vi "Send image to image display controller-subvi.vi"(0 "Image":T1, 1 "Window Title":string, 2 "Window Number":i32, 3 "error in":errorcluster, 4 "Image Type":T2 items=["Grayscale (U8)", "Grayscale (I16)", "Grayscale (SGL)", "Complex (CSG)", "RGB (U32)", "HSL (U32)", "RGB (U64)", "Grayscale (U16)"], 5 "Start display controller?":bool, 6 "Quit display controller?":bool) -> (7 "Image Out":T1, 10 "error out":errorcluster)   [LabVIEW 2014]
doc: "Uses a user event to send an image to Image Display controller which is running in a separate thread, if both Start and Quit inputs are false.\n\nStart = TRUE launches the display controller as a separate thread; all other inputs are ignored.\n\nQuit = TRUE sends a message to the controller telling is to close the display windows and quit."
uses:
  <vilib>/vision/Image Controls.llb/IMAQ Image.ctl
  ctt's/Image to Display event.ctt
  Globals/Initilize Globals.vi
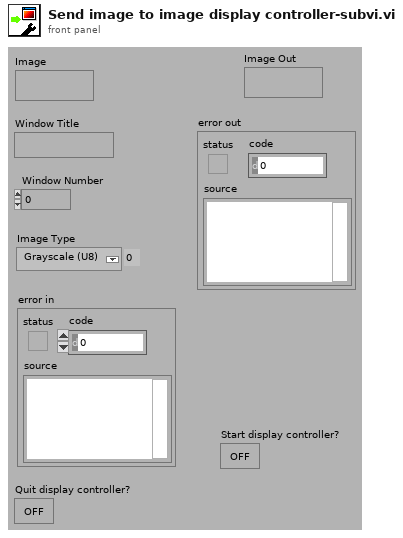
[diagram p1: front panel]
types:
  T1 = typedef "IMAQ Image.ctl" = refnum<image>
  T2 = typedef "Image Type" = u32
  T3 = typedef "Image to Display event.ctt" = cluster{"Image":T1, "Window Title":string, "Window Number":i32, "Image Type":T2, "Quit display controller?":bool}
  T4 = enum32{"Invalid", "Standard", "Closed", "Hidden", "Minimized", "Maximized"}
  T5 = enum32{"Bad", "Idle", "Run top level", "Running"}
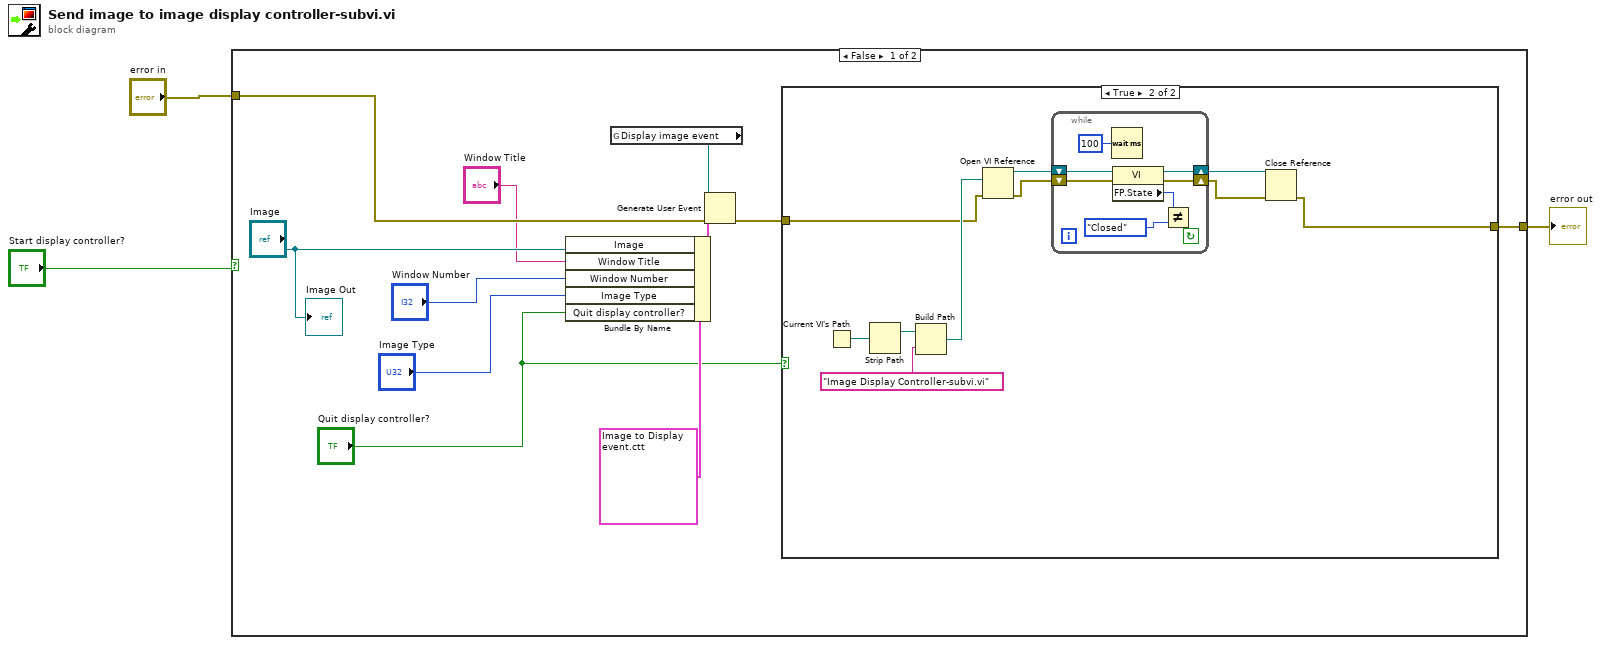
[diagram p0: block diagram]
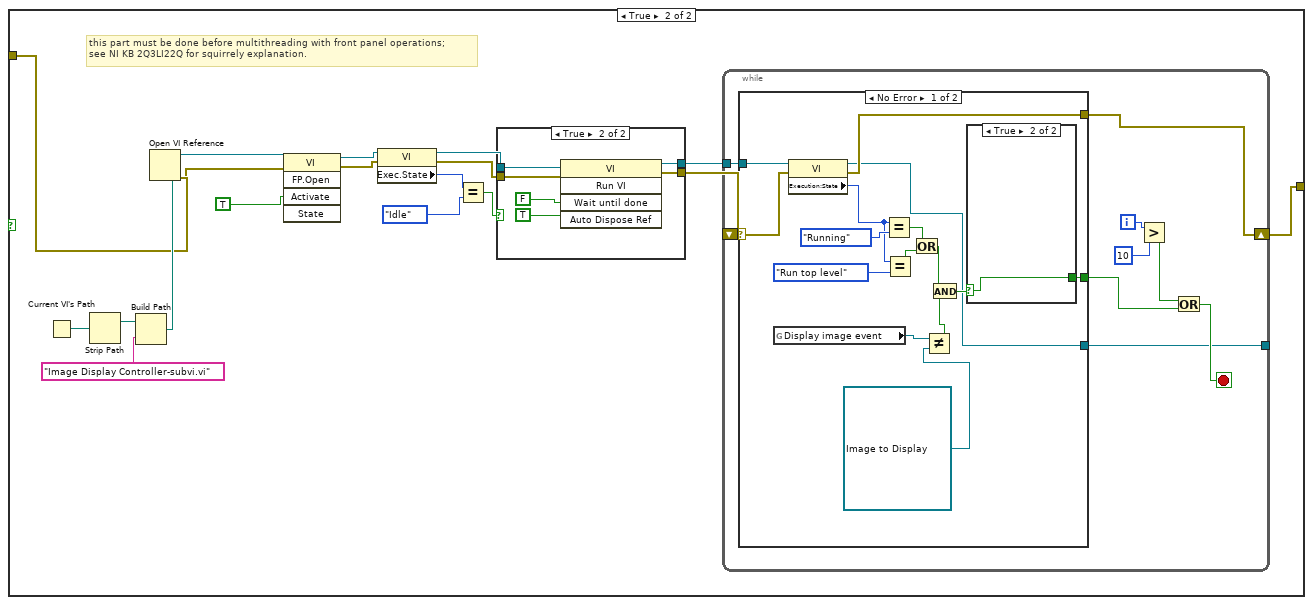
[diagram p3: hidden frame]
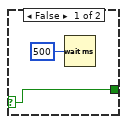
[diagram p5: hidden frame]
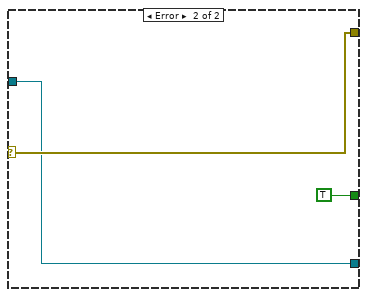
[diagram p6: hidden frame]
diagram:
  n1 = case shown="False" "Start display controller?" {
    tunnel: [w4 w46] -> w3
    tunnel: "error in" -> [w13 w47]
    frame False {
      n2 = Bundle By Name(cluster=T3 {"Image"=refnum, "Window Title"="", "Window Number"=0, "Image Type"=0, "Quit display controller?"=FALSE} ("event data"), "Image"="Image", "Window Title"="Window Title", "Window Number"="Window Number", "Image Type"="Image Type", "Quit display controller?"="Quit display controller?") -> (w10:T3)
      n3 = global read "Initilize Globals.vi" "Display image event"() -> (w12:refnum<user-event>)
      n4 = Generate User Event(user event=w12, event data cluster=w10, error in=w13) -> (error out=w6:errorcluster)  [unwired: 1 in, 1 out]
      n5 = case shown="True" "Quit display controller?" {
        tunnel: w6 -> [w15 w19]
        tunnel: [w15 w16] -> w4
        frame False {
        }
        frame True {
          n6 = Current VI's Path() -> (path=w21:path)
          n7 = Strip Path(path=w21) -> (stripped path=w20:path)  [unwired: 1 out]
          n8 = Build Path(base path=w20, name or relative path="Image Display Controller-subvi.vi") -> (appended path=w23:path)
          n9 = Open VI Reference(vi path=w23, error in (no error)=w19) -> (vi reference=w25:refnum<vi>, error out=w24:errorcluster)  [unwired: 4 out]
          n10 = while {
            shift-right: [w32] -> w18
            shift-left: w25 -> [w30]
            shift-right: [w31] -> w17
            shift-left: w24 -> [w29]
            stop <- w26 continue-if-true
            n11 = Wait (ms)(milliseconds to wait=u32 100) -> ()  [unwired: 1 out]
            n12 = property class="VI"(reference=w30, error in=w29) -> (reference out=w32:refnum<vi>, error out=w31:errorcluster, "FP.State"=w28:T4)
            n13 = Not Equal?(x=w28, y=T4."Closed" ("Front Panel Window:State")) -> (x != y?=w26:bool)
          }
          n14 = Close Reference(reference=w18, error in (no error)=w17) -> (error out=w16:errorcluster)
        }
      }
      "Image Out" <- "Image"
    }
    frame True {
      # "this part must be done before multithreading with front panel operations;\nsee NI KB 2Q3LI22Q for squirrely explanation."
      n15 = Current VI's Path() -> (path=w49:path)
      n16 = Strip Path(path=w49) -> (stripped path=w48:path)  [unwired: 1 out]
      n17 = Build Path(base path=w48, name or relative path="Image Display Controller-subvi.vi") -> (appended path=w51:path)
      n18 = Open VI Reference(vi path=w51, error in (no error)=w47) -> (vi reference=w42:refnum<vi>, error out=w43:errorcluster)  [unwired: 4 out]
      n19 = invoke class="VI" method="FP.Open"(reference=w42, error in=w43, "Activate"=TRUE ("Front Panel Window:Open")) -> (reference out=w40:refnum<vi>, error out=w39:errorcluster)  [unwired: 2 in, 3 out]
      n20 = property class="VI"(reference=w40, error in=w39) -> (reference out=w34:refnum<vi>, error out=w35:errorcluster, "Exec.State"=w38:T5)
      n21 = Equal?(x=w38, y=T5."Idle" ("Execution:State")) -> (x = y?=w36:bool)
      n22 = case shown="True" w36 {
        tunnel: [w53 w58] -> w45
        tunnel: [w52 w57] -> w44
        tunnel: w34 -> [w53 w55]
        tunnel: w35 -> [w52 w54]
        frame False {
        }
        frame True {
          n23 = invoke class="VI" method="Run VI"(reference=w55, error in=w54, "Wait until done"=FALSE, "Auto Dispose Ref"=TRUE ("Wait until done")) -> (reference out=w58:refnum<vi>, error out=w57:errorcluster)  [unwired: 1 in, 3 out]
        }
      }
      n24 = while {
        tunnel: w45 -> [w68]
        shift-right: [w60] -> w46
        shift-left: w44 -> [w67]
        tunnel: [w62] -> _
        i -> [w66]
        stop <- w63 stop-if-true
        n25 = case shown="No Error" w67 {
          selector: w67 -> [w72 w88]
          tunnel: w68 -> [w75 w87]
          tunnel: [w73 TRUE] -> w64
          tunnel: [w71 w88] -> w60
          tunnel: [w70 w87] -> w62
          frame No Error {
            n26 = global read "Initilize Globals.vi" "Display image event"() -> (w81:refnum<user-event>)
            n27 = property class="VI"(reference=w75, error in=w72) -> (reference out=w70:refnum<vi>, error out=w71:errorcluster, "Execution:State"=w76:T5)
            n28 = Equal?(x=w76, y=T5."Running" ("Execution:State")) -> (x = y?=w80:bool)
            n29 = Equal?(x=w76, y=T5."Run top level" ("Execution:State")) -> (x = y?=w79:bool)
            n30 = Or(x=w80, y=w79) -> (x .or. y?=w82:bool)
            n31 = Not Equal?(x=w81, y=refnum<user-event> refnum ("Display image event")) -> (x != y?=w83:bool)
            n32 = And(x=w82, y=w83) -> (x .and. y?=w74:bool)
            n33 = case shown="True" w74 {
              selector: w74 -> [w84 w86]
              tunnel: [w84 w86] -> w73
              frame False {
                n34 = Wait (ms)(milliseconds to wait=u32 500) -> ()  [unwired: 1 out]
              }
              frame True {
              }
            }
          }
          frame Error {
          }
        }
        n35 = Greater?(x=w66, y=10) -> (0:w61:bool)
        n36 = Or(x=w61, y=w64) -> (x .or. y?=w63:bool)
      }
    }
  }
  "error out" <- w3
